vi "Update Inst Studio Connected Status.vi"(8 "error in (no error)":errorcluster, 11 "CIF_UI in":refnum<class "CIF_UI.lvclass">) -> (0 "error out":errorcluster)   [LabVIEW 2021, in "CIF_UI.lvclass"]
uses:
  CIF_UI.lvclass
  CIF_UI.lvclass/CIF_UI.ctl
  Instrument Studio/PluginSDK/Plugin Session.lvclass
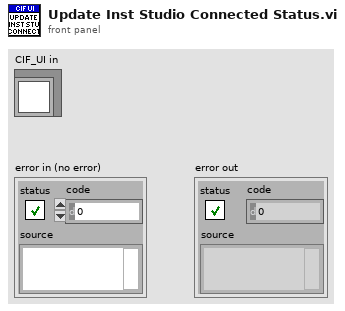
[diagram p1: front panel]
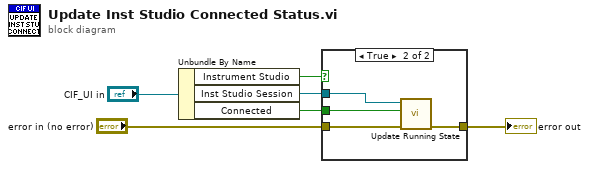
[diagram p0: block diagram]
diagram:
  n1 = Unbundle By Name("CIF_UI in") -> ("Instrument Studio"=w5:bool, "Inst Studio Session"=w4:refnum<class "Plugin Session.lvclass">, "Connected"=w3:bool)
  n2 = case shown="True" w5 {
    tunnel: [w7 w11] -> w6
    tunnel: w4 -> [_ w10]
    tunnel: w3 -> [_ w9]
    tunnel: "error in (no error)" -> [w7 w8]
    frame False {
    }
    frame True {
      n3 = call "Update Running State.vi"("error in (no error)"=w8, "Is Running"=w9, "Plugin Session in"=w10) -> ("error out"=w11:errorcluster)  [unwired: 7 in, 1 out]
    }
  }
  "error out" <- w6
